vi "Connection Info.vi"(10 "路径":path) -> (2 "Connection Info":string)   [LabVIEW 2019]
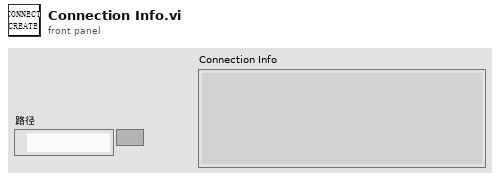
[diagram p1: front panel]
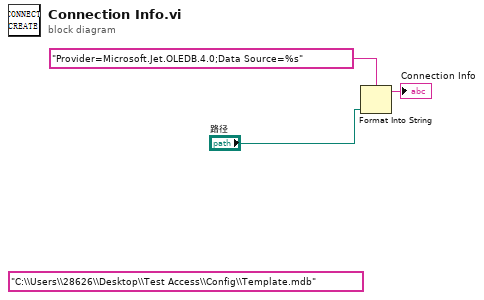
[diagram p0: block diagram]
diagram:
  (unwired) "C:\\Users\\28626\\Desktop\\Test Access\\Config\\Template.mdb" ("输入 1")
  n1 = Format Into String(format string="Provider=Microsoft.Jet.OLEDB.4.0;Data Source=%s" ("格式字符串"), "路径") -> (resulting string=→"Connection Info":string)  [unwired: 2 in, 1 out]
